vi "Velocity _Motor_Pid.vi"(10 "swerve mod":i32, 11 "MotorControlDevRef":T1) -> ()   [LabVIEW 2020]
uses:
  <vilib>/Rock Robotics/WPI/MotorControl/WPI_MotorControlDeviceRef.ctl
  <vilib>/Rock Robotics/WPI/MotorControl/WPI_MotorControlType.ctl
  <vilib>/Rock Robotics/SystemInterfaces/DIO/FPGA_DIOPWMChannel.ctl
  <vilib>/Rock Robotics/WPI/PWM/WPI_PWMDeadband.ctl
  <vilib>/Rock Robotics/SystemInterfaces/DIO/FPGA_DIOChannel.ctl
  Robot Global Data.vi
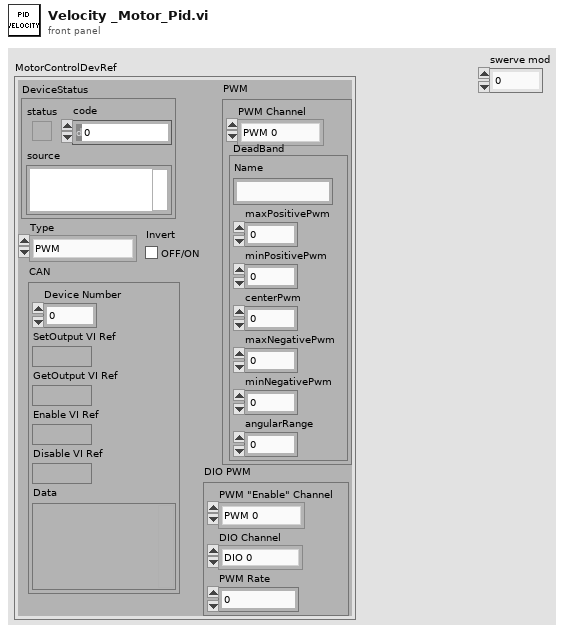
[diagram p1: front panel]
types:
  T1 = typedef "WPI_MotorControlDeviceRef.ctl" = cluster{"DeviceStatus":errorcluster, "Type":T2, "PWM":cluster{"PWM Channel":T3, "DeadBand":T4}, "CAN":cluster{"Device Number":u8, "SetOutput VI Ref":variant, "GetOutput VI Ref":variant, "Enable VI Ref":variant, "Disable VI Ref":variant, "Data":variant}, "Invert":bool, "DIO PWM":cluster{"PWM \"Enable\" Channel":T3, "DIOChannel":T5, "PWM Rate":dbl}}
  T2 = typedef "WPI_MotorControlType.ctl" = enum16{"PWM", "CAN", "DIO PWM"}
  T3 = typedef "FPGA_DIOPWMChannel.ctl" = enum8{"PWM 0", "PWM 1", "PWM 2", "PWM 3", "PWM 4", "PWM 5", "PWM 6", "PWM 7", "PWM 8", "PWM 9", "PWM MXP 0", "PWM MXP 1", "PWM MXP 2", "PWM MXP 3", "PWM MXP 4", "PWM MXP 5", "PWM MXP 6", "PWM MXP 7", "PWM MXP 8", "PWM MXP 9", "Invalid"}
  T4 = typedef "WPI_PWMDeadband.ctl" = cluster{"Name":string, "maxPositivePwm":i32, "minPositivePwm":i32, "centerPwm":i32, "maxNegativePwm":i32, "minNegativePwm":i32, "angularRange":u16}
  T5 = typedef "FPGA_DIOChannel.ctl" = enum8{"DIO 0", "DIO 1", "DIO 2", "DIO 3", "DIO 4", "DIO 5", "DIO 6", "DIO 7", "DIO 8", "DIO 9", "DIO MXP 0", "DIO MXP 1", "DIO MXP 2", "DIO MXP 3", "DIO MXP 4", "DIO MXP 5", "DIO MXP 6", "DIO MXP 7", "DIO MXP 8", "DIO MXP 9", "DIO MXP 10", "DIO MXP 11", "DIO MXP 12", "DIO MXP 13", "DIO MXP 14", "DIO MXP 15", "SPI Port CS1", "SPI Port CS2", "SPI Port CS3", "SPI Port MISO", "SPI Port MOSI", "Invalid"}
  T6 = typedef "Trajectory_Library.lvlib/SWERVE_DRIVE_MODULE_STATE.ctl" = cluster{"Speed":dbl, "Angle":T7}
  T7 = typedef "Trajectory_Library.lvlib/ROTATION2D.ctl" = cluster{"VALUE":dbl, "COS":dbl, "SIN":dbl}
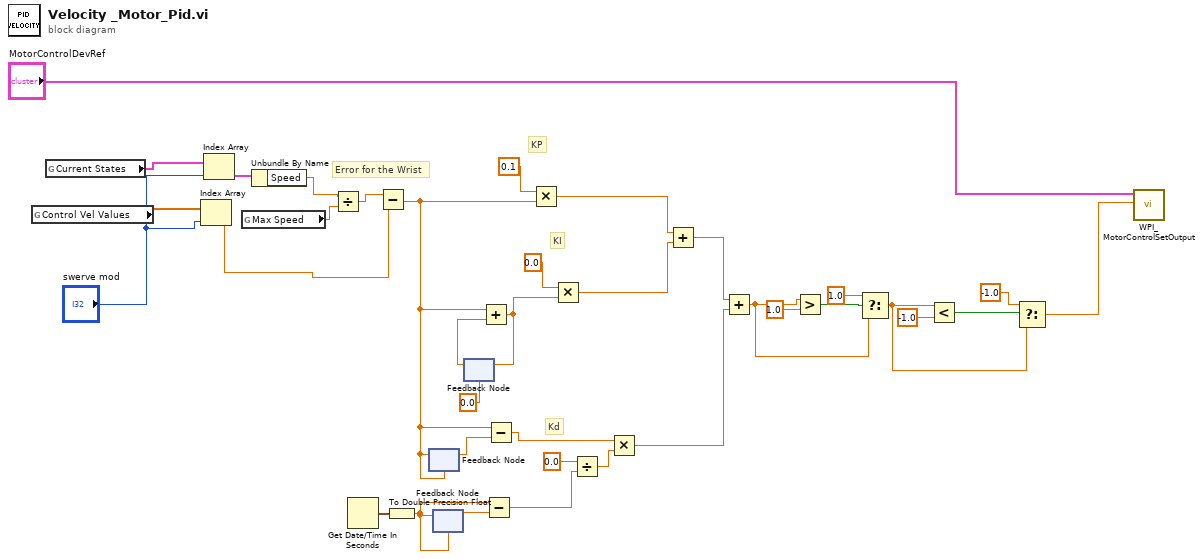
[diagram p0: block diagram]
diagram:
  # "Kd"
  # "KI"
  # "Error for the Wrist"
  # "KP"
  n1 = global read "Robot Global Data.vi" "Control Vel Values"() -> (w36:dbl[])
  n2 = global read "Robot Global Data.vi" "Current States"() -> (w34:T6[])
  n3 = Index Array(array=w36, index="swerve mod") -> (element=w4:dbl)
  n4 = Index Array(array=w34, index="swerve mod") -> (element=w35:T6)
  n5 = global read "Robot Global Data.vi" "Max Speed"() -> (w2:dbl)
  n6 = Unbundle By Name(w35) -> ("Speed"=w3:dbl)
  n7 = Divide(x=w3, y=w2) -> (x/y=w1:dbl)
  n8 = Get Date/Time In Seconds() -> (seconds since 1Jan1904=w20:timestamp)
  n9 = Subtract(x=w1, y=w4) -> (x-y=w32:dbl)
  n10 = To Double Precision Float(number=w20) -> (double precision float=w22:dbl)
  n11 = feedback #1(w32) -> (w29:dbl)
  n12 = feedback-in #1(w32) -> ()
  n13 = feedback #2(w22) -> (w21:dbl)
  n14 = feedback-in #2(w22) -> ()
  n15 = feedback #3(0.0) -> (w16:dbl)
  n16 = Add(x=w32, y=w16) -> (x+y=w19:dbl)
  n17 = feedback-in #3(w19) -> ()
  n18 = Subtract(x=w22, y=w21) -> (x-y=w30:dbl)
  n19 = Subtract(x=w32, y=w29) -> (x-y=w28:dbl)
  n20 = Multiply(x=0.1 ("y"), y=w32) -> (x*y=w26:dbl)
  n21 = Multiply(x=0.0 ("y"), y=w19) -> (x*y=w24:dbl)
  n22 = Divide(x=0.0, y=w30) -> (x/y=w31:dbl)
  n23 = Multiply(x=w28, y=w31) -> (x*y=w25:dbl)
  n24 = Add(x=w26, y=w24) -> (x+y=w27:dbl)
  n25 = Add(x=w27, y=w25) -> (x+y=w11:dbl)
  n26 = Greater?(x=w11, y=1.0) -> (0:w13:bool)
  n27 = Select(t=1.0, s=w13, f=w11) -> (s? t:f=w7:dbl)
  n28 = Less?(x=w7, y=-1.0) -> (x < y?=w9:bool)
  n29 = Select(t=-1.0, s=w9, f=w7) -> (s? t:f=w6:dbl)
  n30 = call <vilib>:"WPI_MotorControlSetOutput.vi"("Output"=w6, "MotorControlDevRef"="MotorControlDevRef") -> ()  [unwired: 7 in, 3 out]
